vi "area-and-perimeter.vi"() -> ()   [LabVIEW 2025]
panel:
  in  "value of r2":dbl
  out "area":dbl
  out "perim":dbl
  in  "value of r":dbl
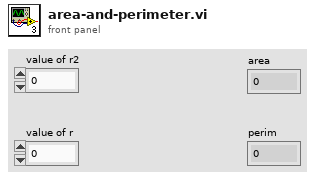
[diagram p1: front panel]
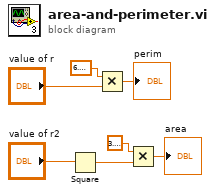
[diagram p0: block diagram]
diagram:
  n1 = Square(x="value of r2") -> (x^2=w3:dbl)
  n2 = Multiply(x=6.283185307179586, y="value of r") -> (x*y=→"perim":dbl)
  n3 = Multiply(x=3.141592653589793, y=w3) -> (x*y=→"area":dbl)
